vi "题目5.vi"() -> ()   [LabVIEW 2017]
panel:
  in  "停止":bool
  in  "分数":dbl
  out "恭喜":bool
  out "通过":bool
  out "警告":bool
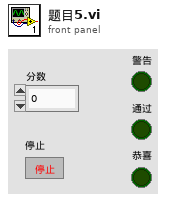
[diagram p1: front panel]
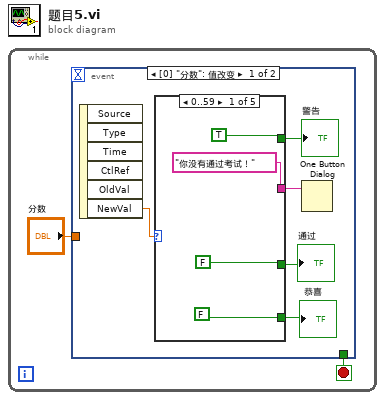
[diagram p0: block diagram]
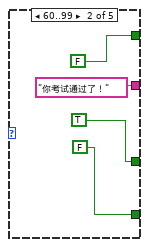
[diagram p2: hidden frame]
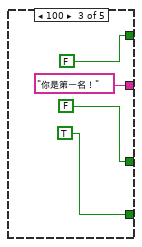
[diagram p3: hidden frame]
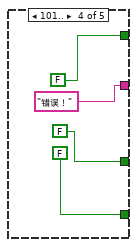
[diagram p4: hidden frame]
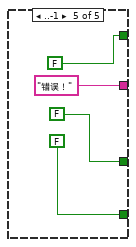
[diagram p5: hidden frame]
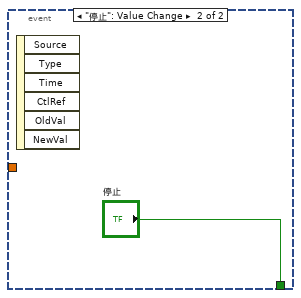
[diagram p6: hidden frame]
diagram:
  n1 = while {
    stop <- w1 stop-if-true
    n2 = event shown="[0] \"分数\": 值改变" {
      selector: _ -> [_ _]
      dyn-events: _ -> [_ _]
      timeout: _ -> [_ _]
      tunnel: "分数" -> [_ _]
      tunnel: [_ "停止"] -> w1
      event "分数": Value Change {
        n3 = event-data() -> ("NewVal"=w3:dbl)  [unwired: 1 in, 5 out]
        n4 = case shown="0..59" w3 {
          tunnel: [TRUE FALSE FALSE FALSE FALSE] -> w7
          tunnel: [FALSE TRUE FALSE FALSE FALSE] -> w6
          tunnel: [FALSE FALSE TRUE FALSE FALSE] -> w5
          tunnel: ["你没有通过考试！" "你考试通过了！" "你是第一名！" "错误！" "错误！"] -> w4
          frame 0..59 {
          }
          frame 60..99 {
          }
          frame 100 {
          }
          frame 101.. {
          }
          frame ..-1 {
          }
        }
        "警告" <- w7
        "通过" <- w6
        "恭喜" <- w5
        n5 = One Button Dialog(message=w4) -> ()  [unwired: 1 in, 1 out]
      }
      event "停止": Value Change {
        n6 = event-data() -> ()  [unwired: 1 in, 6 out]
      }
    }
  }
